vi "Open Left Side.vi"(8 "error in (no error)":errorcluster, 11 "This VI":refnum<vi>) -> (0 "error out":errorcluster)   [LabVIEW 2014]
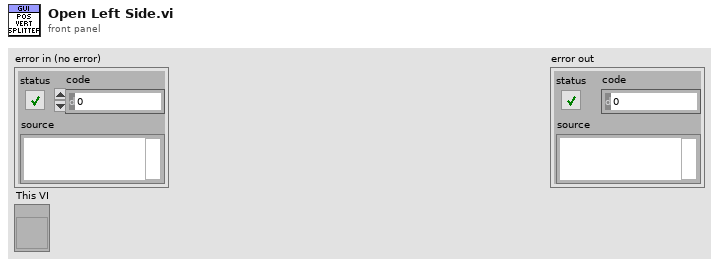
[diagram p1: front panel]
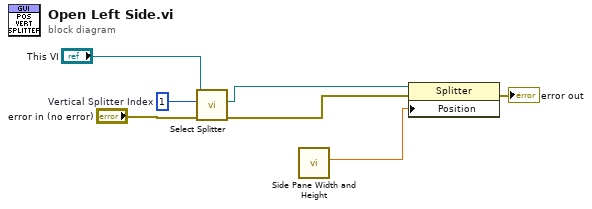
[diagram p0: block diagram]
diagram:
  w5 = 1  # Vertical Splitter Index
  n1 = call "Select Splitter.vi"("error in (no error)"="error in (no error)", "Pane Index"=w5, "This VI"="This VI") -> ("error out"=w1:errorcluster, "Splitter"=w4:refnum<vi>)  [unwired: 6 in, 1 out]
  n2 = call "Side Pane Width and Height.vi"() -> ("Width"=w2:dbl)  [unwired: 9 in, 2 out]
  n3 = property class="Splitter"(reference=w4, error in=w1, "Position"=w2) -> (error out=→"error out":errorcluster)  [unwired: 1 out]
